vi "Error-Save Errors to List.vi"(0 "Codes":i32[](array[numeric]), 5 "Errors":T1(array[cluster])) -> (15 "error out":errorcluster)   [LabVIEW 2020]
uses:
  <vilib>/Utility/config.llb/Write Key (String).vi
  <vilib>/Utility/config.llb/NI_LVConfig.lvlib
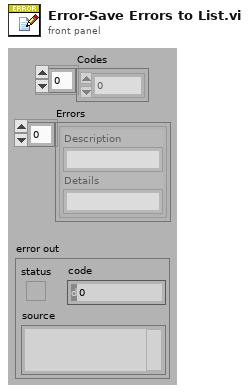
[diagram p1: front panel]
types:
  T1 = cluster{"Description":string, "Details":string}[]
  T2 = typedef "NI_LVConfig.lvlib/Config Data RefNum.ctl" = refnum<k1>
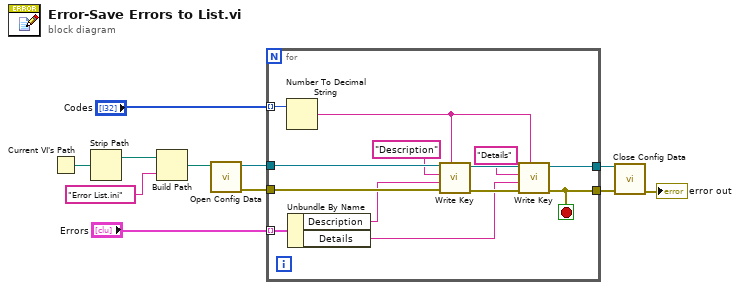
[diagram p0: block diagram]
diagram:
  n1 = Current VI's Path() -> (path=w8:path)
  n2 = Strip Path(path=w8) -> (stripped path=w9:path)  [unwired: 1 out]
  n3 = Build Path(base path=w9, name or relative path="Error List.ini") -> (appended path=w11:path)
  n4 = call <vilib>:"Open Config Data.vi"("configuration file path"=w11) -> ("error out"=w3:errorcluster, "refnum"=w2:T2)  [unwired: 8 in, 1 out]
  n5 = for {
    tunnel: w2 -> [w24]
    tunnel: [w18] -> w6
    tunnel: w3 -> [w19]
    tunnel: [w17] -> w7
    tunnel: "Codes" -> [w16] mode=indexing
    tunnel: "Errors" -> [w14] mode=indexing
    stop <- w18 stop-if-true
    n6 = Number To Decimal String(number=w16) -> (decimal integer string=w15:string)  [unwired: 1 in]
    n7 = Unbundle By Name(w14) -> ("Description"=w13:string, "Details"=w12:string)
    n8 = call-poly <vilib>:"Write Key.vi"("section"=w15, "error in (no error)"=w19, "value"=w13, "key"="Description", "refnum"=w24) -> ("error out"=w21:errorcluster, "refnum out"=w22:T2)  [unwired: 4 in, 1 out]
    n9 = call-poly <vilib>:"Write Key.vi"("section"=w15, "error in (no error)"=w21, "value"=w12, "key"="Details", "refnum"=w22) -> ("error out"=w18:errorcluster, "refnum out"=w17:T2)  [unwired: 4 in, 1 out]
  }
  n10 = call <vilib>:"Close Config Data.vi"("error in (no error)"=w6, "refnum"=w7) -> ("error out"=→"error out":errorcluster)  [unwired: 8 in, 1 out]
